vi "Periodic Tasks.vi"(8 "error in":errorcluster) -> ()   [LabVIEW 2018]
doc: "This VI runs in parallel to other robot code. It can contain as many user-defined periodic loops as you need. These can carry out PID or other sorts of timed response."
panel:
  in  "Seconds from neutral to full (0)":sgl=0.08
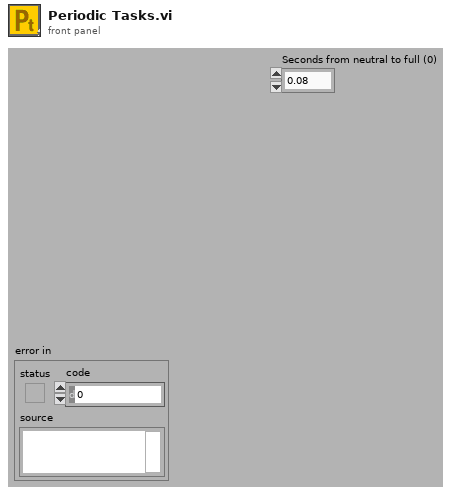
[diagram p1: front panel]
types:
  T1 = typedef "SPARKMAX6Motor.ctl" = cluster{"FrontLeftMaster":T2, "FrontLeftSlave1":T2, "FrontLeftSlave2":T2, "FrontRightMaster":T2, "FrontRightSlave1":T2, "FrontRightSlave2":T2}
  T2 = typedef "WPI_MotorControlDeviceRef.ctl" = cluster{"DeviceStatus":errorcluster, "Type":T3, "PWM":cluster{"PWM Channel":T4, "DeadBand":T5}, "CAN":cluster{"Device Number":u8, "SetOutput VI Ref":variant, "GetOutput VI Ref":variant, "Enable VI Ref":variant, "Disable VI Ref":variant, "Data":variant}, "Invert":bool, "DIO PWM":cluster{"PWM \"Enable\" Channel":T4, "DIOChannel":T6, "PWM Rate":dbl}}
  T3 = typedef "WPI_MotorControlType.ctl" = enum16{"PWM", "CAN", "DIO PWM"}
  T4 = typedef "FPGA_DIOPWMChannel.ctl" = enum8{"PWM 0", "PWM 1", "PWM 2", "PWM 3", "PWM 4", "PWM 5", "PWM 6", "PWM 7", "PWM 8", "PWM 9", "PWM MXP 0", "PWM MXP 1", "PWM MXP 2", "PWM MXP 3", "PWM MXP 4", "PWM MXP 5", "PWM MXP 6", "PWM MXP 7", "PWM MXP 8", "PWM MXP 9", "Invalid"}
  T5 = typedef "WPI_PWMDeadband.ctl" = cluster{"Name":string, "maxPositivePwm":i32, "minPositivePwm":i32, "centerPwm":i32, "maxNegativePwm":i32, "minNegativePwm":i32, "angularRange":u16}
  T6 = typedef "FPGA_DIOChannel.ctl" = enum8{"DIO 0", "DIO 1", "DIO 2", "DIO 3", "DIO 4", "DIO 5", "DIO 6", "DIO 7", "DIO 8", "DIO 9", "DIO MXP 0", "DIO MXP 1", "DIO MXP 2", "DIO MXP 3", "DIO MXP 4", "DIO MXP 5", "DIO MXP 6", "DIO MXP 7", "DIO MXP 8", "DIO MXP 9", "DIO MXP 10", "DIO MXP 11", "DIO MXP 12", "DIO MXP 13", "DIO MXP 14", "DIO MXP 15", "SPI Port CS1", "SPI Port CS2", "SPI Port CS3", "SPI Port MISO", "SPI Port MOSI", "Invalid"}
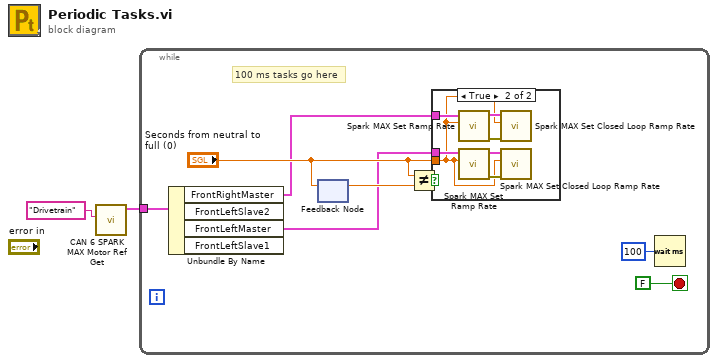
[diagram p0: block diagram]
diagram:
  n1 = call "CAN 6 SPARK MAX Motor Ref Get.vi"("refnum name"="Drivetrain") -> ("TalonSRX6MotorRef out"=w1:T1)  [unwired: 9 in, 1 out]
  n2 = while {
    tunnel: w1 -> [w8]
    stop <- FALSE stop-if-true
    # "100 ms tasks go here"
    n3 = Unbundle By Name(w8) -> ("FrontRightMaster"=w3:T2, "FrontLeftMaster"=w4:T2)  [unwired: 2 out]
    n4 = feedback-in #1("Seconds from neutral to full (0)") -> ()
    n5 = feedback #1() -> (w6:sgl)  [unwired: 1 in]
    n6 = Not Equal?(x="Seconds from neutral to full (0)", y=w6) -> (x != y?=w7:bool)
    n7 = case shown="True" w7 {
      tunnel: w3 -> [_ w17]
      tunnel: w4 -> [_ w16]
      tunnel: "Seconds from neutral to full (0)" -> [_ w11]
      frame False {
      }
      frame True {
        n8 = call <vilib>:"Spark MAX Set Ramp Rate.vi"("Seconds from neutral to full (0)"=w11, "MotorControlDeviceRef in"=w17) -> ("error out"=w14:errorcluster, "MotorControlDeviceRef"=w15:T2)  [unwired: 8 in]
        n9 = call <vilib>:"Spark MAX Set Ramp Rate.vi"("Seconds from neutral to full (0)"=w11, "MotorControlDeviceRef in"=w16) -> ("error out"=w12:errorcluster, "MotorControlDeviceRef"=w13:T2)  [unwired: 8 in]
        n10 = call <vilib>:"Spark MAX Set Closed Loop Ramp Rate.vi"("error in (no error)"=w14, "Seconds from neutral to full (0)"=w11, "MotorControlDeviceRef in"=w15) -> ()  [unwired: 7 in, 2 out]
        n11 = call <vilib>:"Spark MAX Set Closed Loop Ramp Rate.vi"("error in (no error)"=w12, "Seconds from neutral to full (0)"=w11, "MotorControlDeviceRef in"=w13) -> ()  [unwired: 7 in, 2 out]
      }
    }
    n12 = Wait (ms)(milliseconds to wait=u32 100) -> ()  [unwired: 1 out]
  }
